vi "Convert text settings to settable cluster.vi"(1 "cluster from Get Settings":T2) -> (0 "cluster for Set Font":T1)   [LabVIEW 2017, in "NI_ReportGenerationCore.lvlib"]
doc: "Converts text settings output of 'Get Report Settings' to text settings input for 'Set Report Font.'\nThis function is useful when getting the current settings, changing settings, and restoring them."
uses:
  <vilib>/Utility/NIReport.llb/NI_ReportGenerationCore.lvlib
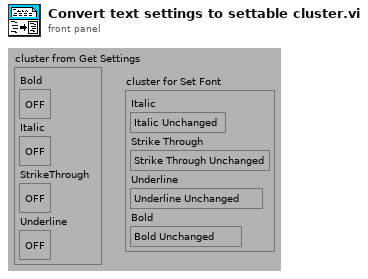
[diagram p1: front panel]
types:
  T1 = cluster{"Italic":enum16{"Italic Unchanged", "Italic On", "Italic Off"}, "Strike Through":enum16{"Strike Through Unchanged", "Strike Through On", "Strike Through Off"}, "Underline":enum16{"Underline Unchanged", "Underline On", "Underline Off"}, "Bold":enum16{"Bold Unchanged", "Bold On", "Bold Off"}}
  T2 = cluster{"Bold":bool, "Italic":bool, "StrikeThrough":bool, "Underline":bool}
  T3 = enum16{"Italic Unchanged", "Italic On", "Italic Off"}
  T4 = enum16{"Strike Through Unchanged", "Strike Through On", "Strike Through Off"}
  T5 = enum16{"Underline Unchanged", "Underline On", "Underline Off"}
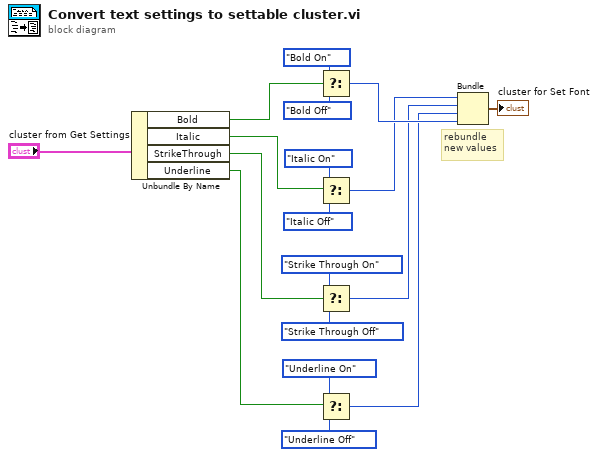
[diagram p0: block diagram]
diagram:
  # "rebundle\nnew values"
  n1 = Unbundle By Name("cluster from Get Settings") -> ("Bold"=w5:bool, "Italic"=w6:bool, "StrikeThrough"=w11:bool, "Underline"=w12:bool)
  n2 = Select(t=enum16{"Bold Unchanged", "Bold On", "Bold Off"}."Bold On" ("Bold"), s=w5, f=enum16{"Bold Unchanged", "Bold On", "Bold Off"}."Bold Off" ("Bold")) -> (s? t:f=w18:enum16{"Bold Unchanged", "Bold On", "Bold Off"})
  n3 = Select(t=T3."Italic On" ("Italic"), s=w6, f=T3."Italic Off" ("Italic")) -> (s? t:f=w15:T3)
  n4 = Select(t=T4."Strike Through On" ("Strike Through"), s=w11, f=T4."Strike Through Off" ("Strike Through")) -> (s? t:f=w16:T4)
  n5 = Select(t=T5."Underline On" ("Underline"), s=w12, f=T5."Underline Off" ("Underline")) -> (s? t:f=w17:T5)
  n6 = Bundle("Italic"=w15, "Strike Through"=w16, "Underline"=w17, "Bold"=w18) -> (→"cluster for Set Font":T1)  [unwired: 1 in]
